vi "engine.prestep.vi"(8 "error in":errorcluster, 10 "clk(NaN)":dbl=nan, 11 "proc in":variant[](array[variant])) -> (0 "error out":errorcluster, 1 "isRunning":bool, 2 "sysClk out":dbl format="%#.1f", 3 "HeaderElement out":cluster{variant[]})   [LabVIEW 2024]
uses:
  controls/typeProcVarientName.ctl
  Polymorphics/variantCtrlBoolean.vi
  Polymorphics/variantCtrlString.vi
  Polymorphics/variantCtrlNumber.vi
  proc.util.validateParamExist.vi
  <vilib>/Utility/error.llb/Clear Errors.vi
  util.error.create.vi
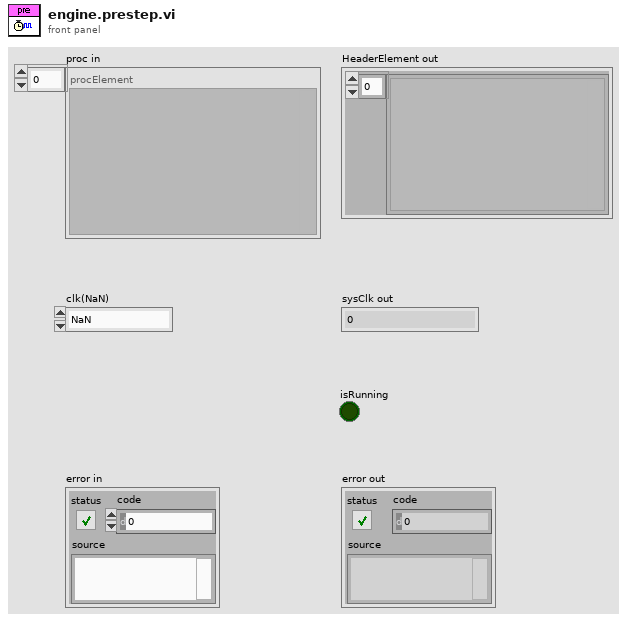
[diagram p1: front panel]
types:
  T1 = typedef "typeProcVarientName.ctl" = enum16{"procNameID", "procModuleID", "procPath", "procIsRunning", "procIndex", "procModule", "procRegisterNumeric", "procRegisterString", "procReport", "procReportPrev", "procCLK", "procStepPointer", "procType"}
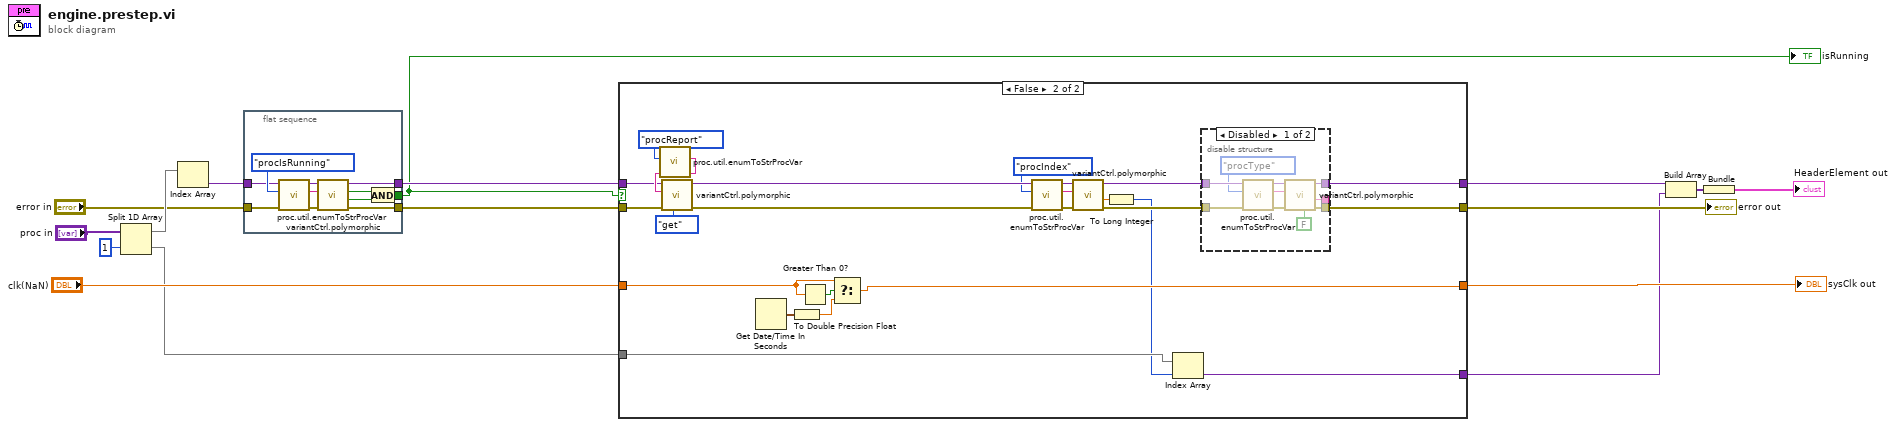
[diagram p0: block diagram]
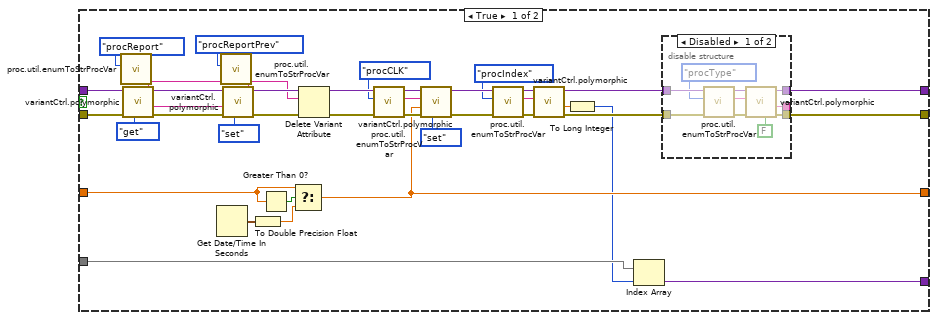
[diagram p2: hidden frame]
diagram:
  n1 = Split 1D Array(array="proc in", index=1) -> (first subarray=w13:variant[], second subarray=w8:variant[])
  n2 = Index Array(array=w13) -> (element=w3:variant)  [unwired: 1 in]
  n3 = flat-sequence {
    tunnel: [w25] -> w2
    tunnel: [w24] -> w4
    tunnel: [w22] -> w1
    tunnel: w3 -> [w18]
    tunnel: "error in" -> [w17]
    frame #0 {
      n4 = call "proc.util.enumToStrProcVar.vi"("Proc var"=typeProcVarientName."procIsRunning") -> ("String"=w20:string)  [unwired: 10 in]
      n5 = call-poly "variantCtrl.polymorphic.vi"("error in"=w17, "name in"=w20, "variant in"=w18) -> ("error out"=w24:errorcluster, "Boolean Value out"=w21:bool, "isFound?"=w23:bool, "variant out"=w25:variant)  [unwired: 5 in]
      n6 = And(x=w23, y=w21) -> (x .and. y?=w22:bool)
    }
  }
  n7 = case shown="False" w1 {
    tunnel: [w60 w92] -> w16
    tunnel: "clk(NaN)" -> [w54 w88]
    tunnel: [w53 w87] -> w11
    tunnel: [w52 w86] -> w10
    tunnel: w8 -> [w51 w85]
    tunnel: [w50 w84] -> w7
    tunnel: w4 -> [w27 w72]
    tunnel: w2 -> [w26 w71]
    frame True {
      n8 = call "proc.util.enumToStrProcVar.vi"("Proc var"=typeProcVarientName."procReport" ("proc var")) -> ("String"=w41:string)  [unwired: 10 in]
      n9 = call-poly "variantCtrl.polymorphic.vi"("menu in (get)"=enum16{"get", "set"}."get", "error in"=w27, "name in"=w41, "Step in"=w26) -> ("error out"=w39:errorcluster, "String Value"=w48:string, "Step out"=w49:variant)  [unwired: 4 in, 1 out]
      n10 = Get Date/Time In Seconds() -> (seconds since 1Jan1904=w56:timestamp)
      n11 = call "proc.util.enumToStrProcVar.vi"("Proc var"=typeProcVarientName."procReportPrev" ("proc var")) -> ("String"=w44:string)  [unwired: 10 in]
      n12 = call-poly "variantCtrl.polymorphic.vi"("menu in (get)"=enum16{"get", "set"}."set", "error in"=w39, "String Value"=w48, "name in"=w44, "Step in"=w49) -> ("error out"=w40:errorcluster, "Step out"=w42:variant)  [unwired: 3 in, 2 out]
      n13 = To Double Precision Float(number=w56) -> (double precision float=w55:dbl)
      n14 = Greater Than 0?(x=w54) -> (x > 0?=w57:bool)
      n15 = Select(t=w54, s=w57, f=w55) -> (s? t:f=w53:dbl)
      n16 = Delete Variant Attribute(4:w40, 6:w41, 7:w42) -> (0:w58:errorcluster, 3:w59:variant)  [unwired: 1 out]
      n17 = call "proc.util.enumToStrProcVar.vi"("Proc var"=typeProcVarientName."procCLK") -> ("String"=w36:string)  [unwired: 10 in]
      n18 = call-poly "variantCtrl.polymorphic.vi"("menu in (get)"=enum16{"get", "set"}."set", "error in"=w58, "number"=w53, "name in"=w36, "variant in"=w59) -> ("error out"=w37:errorcluster, "variant out"=w38:variant)  [unwired: 3 in, 2 out]
      n19 = call "proc.util.enumToStrProcVar.vi"("Proc var"=typeProcVarientName."procIndex") -> ("String"=w29:string)  [unwired: 10 in]
      n20 = call-poly "variantCtrl.polymorphic.vi"("error in"=w37, "name in"=w29, "variant in"=w38) -> ("error out"=w32:errorcluster, "number"=w30:dbl, "variant out"=w33:variant)  [unwired: 5 in, 1 out]
      n21 = To Long Integer(number=w30) -> (32bit integer=w31:i32)
      n22 = Index Array(array=w51, index=w31) -> (element=w50:variant)
      n23 = disable-structure shown="Disabled" {
        disable-tunnel: [w68 w70] -> w52
        disable-tunnel: [w67 w69] -> w60
        disable-tunnel: w33 -> [w66 w70]
        disable-tunnel: w32 -> [w65 w69]
        disable-tunnel: [w62 _] -> _
        frame Disabled {
          n24 = call "proc.util.enumToStrProcVar.vi"("Proc var"=typeProcVarientName."procType") -> ("String"=w63:string)  [unwired: 10 in]
          n25 = call-poly "variantCtrl.polymorphic.vi"("isRequired (T)"=FALSE, "error in"=w65, "name in"=w63, "Step in"=w66) -> ("error out"=w67:errorcluster, "String Value"=w62:string, "Step out"=w68:variant)  [unwired: 4 in, 1 out]
        }
        frame Enabled {
        }
      }
    }
    frame False {
      n26 = call "proc.util.enumToStrProcVar.vi"("Proc var"=typeProcVarientName."procReport" ("proc var")) -> ("String"=w80:string)  [unwired: 10 in]
      n27 = call-poly "variantCtrl.polymorphic.vi"("menu in (get)"=enum16{"get", "set"}."get", "error in"=w72, "name in"=w80, "Step in"=w71) -> ("error out"=w79:errorcluster, "Step out"=w83:variant)  [unwired: 4 in, 2 out]
      n28 = Get Date/Time In Seconds() -> (seconds since 1Jan1904=w90:timestamp)
      n29 = To Double Precision Float(number=w90) -> (double precision float=w89:dbl)
      n30 = Greater Than 0?(x=w88) -> (x > 0?=w91:bool)
      n31 = Select(t=w88, s=w91, f=w89) -> (s? t:f=w87:dbl)
      n32 = call "proc.util.enumToStrProcVar.vi"("Proc var"=typeProcVarientName."procIndex") -> ("String"=w74:string)  [unwired: 10 in]
      n33 = call-poly "variantCtrl.polymorphic.vi"("error in"=w79, "name in"=w74, "variant in"=w83) -> ("error out"=w77:errorcluster, "number"=w75:dbl, "variant out"=w78:variant)  [unwired: 5 in, 1 out]
      n34 = To Long Integer(number=w75) -> (32bit integer=w76:i32)
      n35 = Index Array(array=w85, index=w76) -> (element=w84:variant)
      n36 = disable-structure shown="Disabled" {
        disable-tunnel: [w100 w102] -> w86
        disable-tunnel: [w99 w101] -> w92
        disable-tunnel: w78 -> [w98 w102]
        disable-tunnel: w77 -> [w97 w101]
        disable-tunnel: [w94 _] -> _
        frame Disabled {
          n37 = call "proc.util.enumToStrProcVar.vi"("Proc var"=typeProcVarientName."procType") -> ("String"=w95:string)  [unwired: 10 in]
          n38 = call-poly "variantCtrl.polymorphic.vi"("isRequired (T)"=FALSE, "error in"=w97, "name in"=w95, "Step in"=w98) -> ("error out"=w99:errorcluster, "String Value"=w94:string, "Step out"=w100:variant)  [unwired: 4 in, 1 out]
        }
        frame Enabled {
        }
      }
    }
  }
  "error out" <- w16
  "sysClk out" <- w11
  n39 = Build Array(w10, w7) -> (w9:variant[])
  n40 = Bundle(w9) -> (→"HeaderElement out":cluster{variant[]})  [unwired: 1 in]
  "isRunning" <- w1
